vi "FTW-Container-Support-XML-LVSchemaToIR.vi"(0 "XML Node":refnum<k20>, 5 "Indent Characters":string, 7 "Indent Level":i32=1, 11 "error in":errorcluster) -> (4 "XML Node out":refnum<k20>, 6 "Serialized Node":string, 15 "error out":errorcluster)   [LabVIEW 2013, in "FTW-Container.lvclass"]
uses:
  FTW-Container.lvclass
  <resource>/objmgr/DOMUserDefRef.rc
panel:
  # "Inputs"
  # "Outputs"
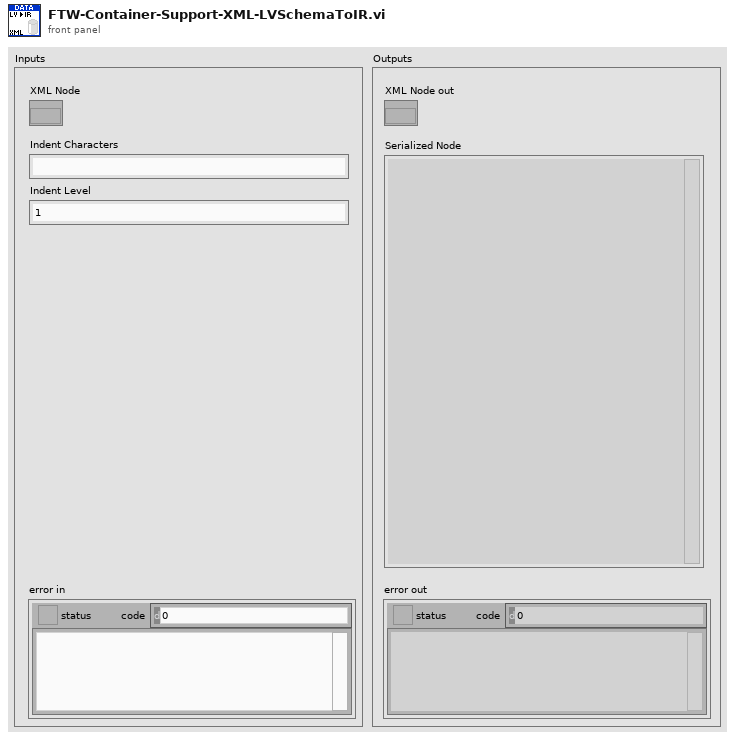
[diagram p1: front panel]
types:
  T1 = typedef "FTW-JSON-Datatype.ctl" = enum16{"Object", "Array", "String", "Number", "Boolean", "NULL", "<Refnum>", "<Enum>", "<Unknown>"}
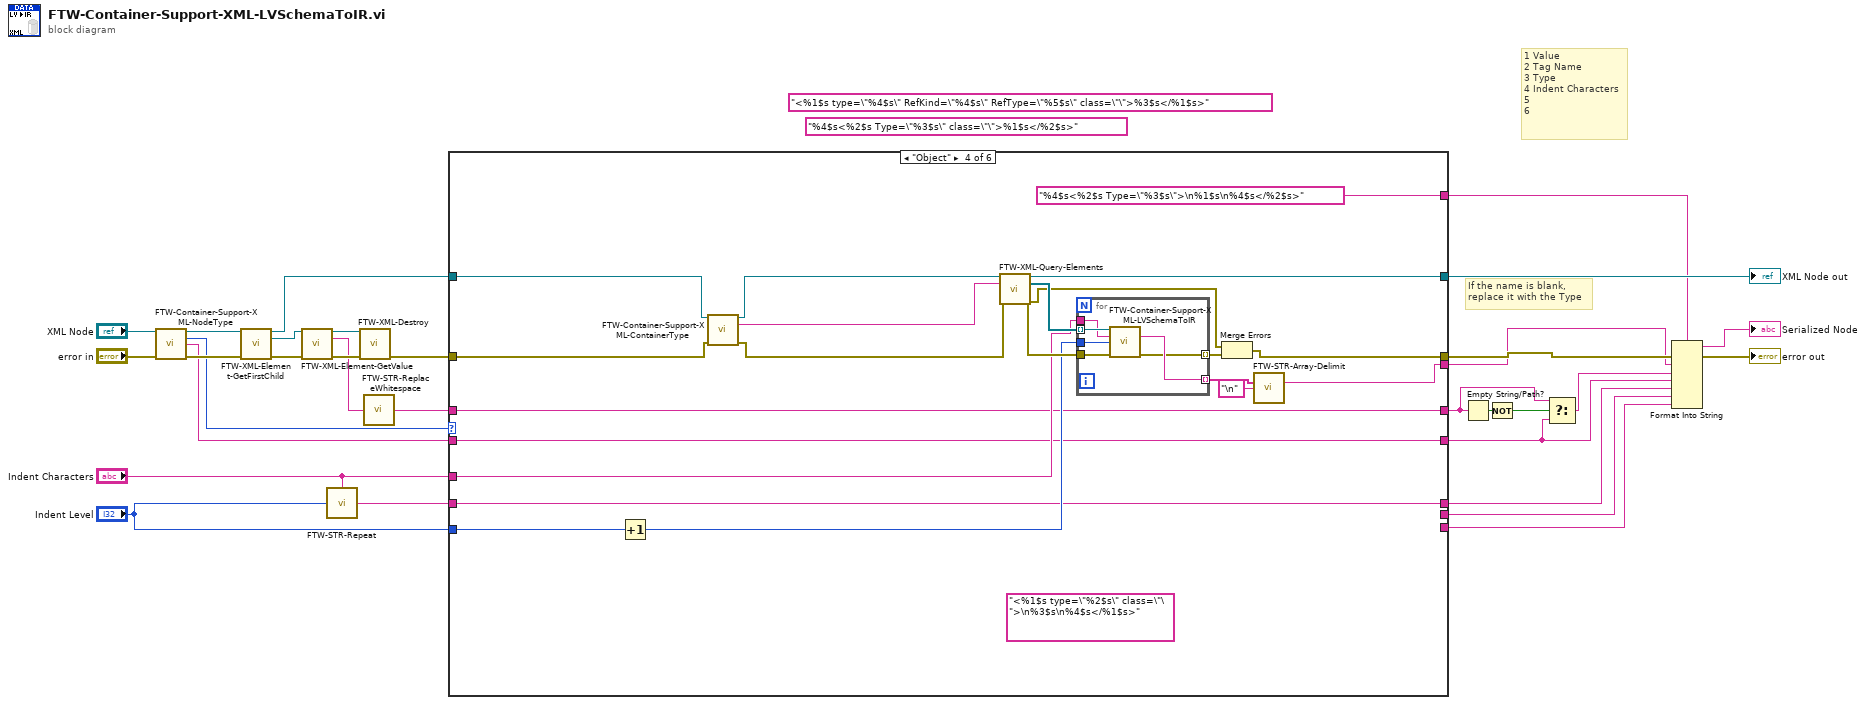
[diagram p0: block diagram]
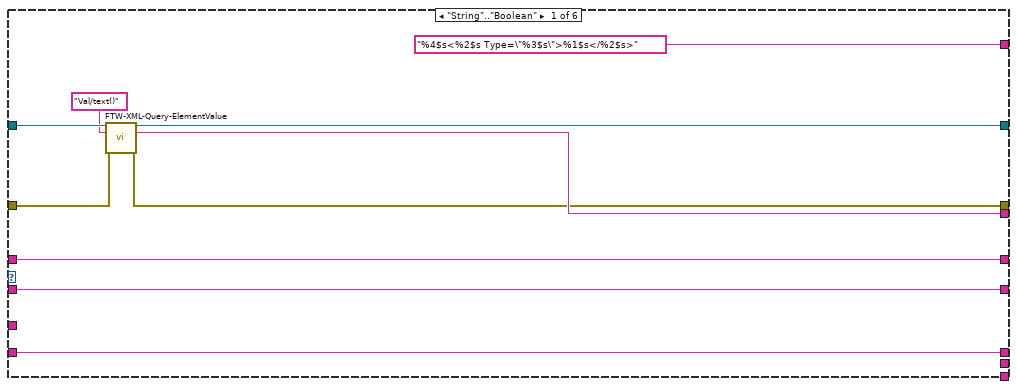
[diagram p2: hidden frame]
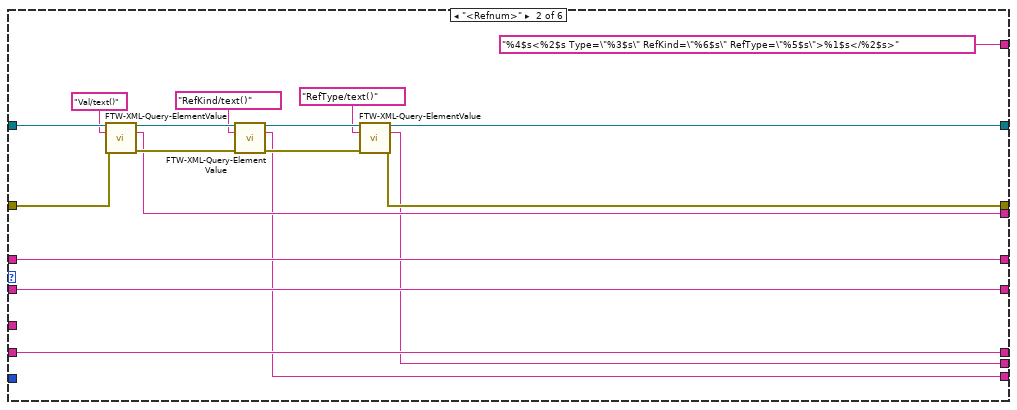
[diagram p3: hidden frame]
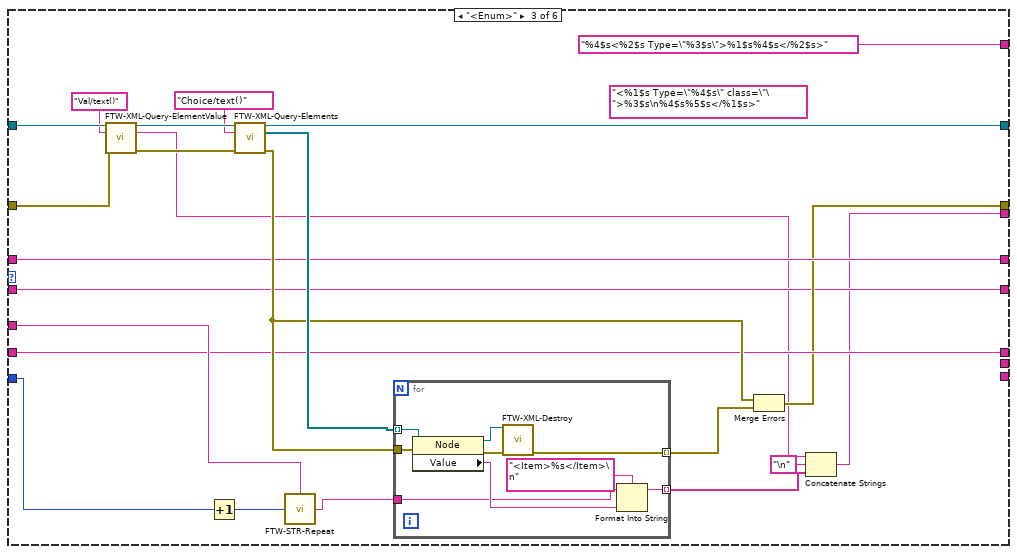
[diagram p4: hidden frame]
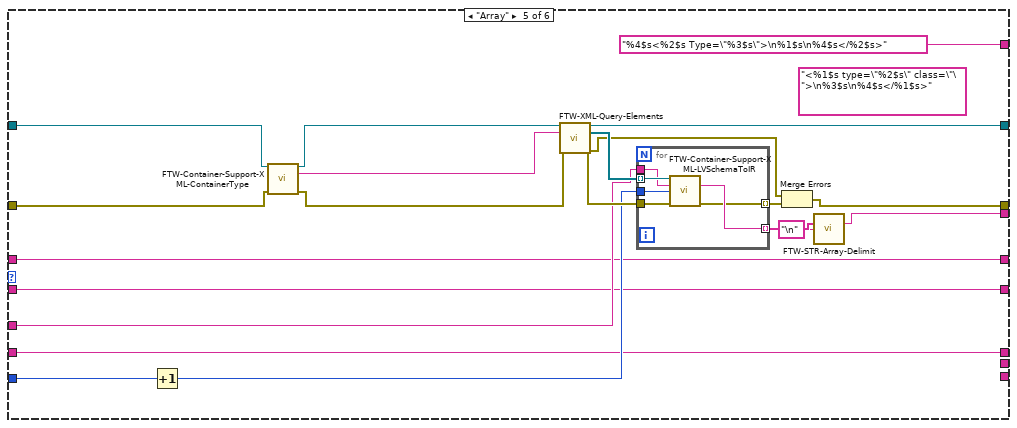
[diagram p5: hidden frame]
diagram:
  (unwired) "%4$s<%2$s Type=\"%3$s\" class=\"\">%1$s</%2$s>"
  (unwired) "<%1$s type=\"%4$s\" RefKind=\"%4$s\" RefType=\"%5$s\" class=\"\">%3$s</%1$s>" ("format string")
  # "If the name is blank,\nreplace it with the Type"
  # "1 Value\n2 Tag Name\n3 Type\n4 Indent Characters\n5\n6"
  n1 = call "FTW-Container-Support-XML-NodeType.vi"("Element Node"="XML Node", "error in"="error in") -> ("Element Node out"=w23:refnum<k20>, "JSON Type"=w20:T1, "Node XML Type"=w12:string, "error out"=w21:errorcluster)  [unwired: 10 in]
  n2 = call "FTW-XML-Element-GetFirstChild.vi"("Element Node"=w23, "error in"=w21) -> ("Element Node out"=w26:refnum<k20>, "First Child Element Node"=w27:refnum<k20>, "error out"=w28:errorcluster)  [unwired: 10 in, 1 out]
  n3 = call "FTW-XML-Element-GetValue.vi"("XML Node"=w27, "error in"=w28) -> ("XML Node out"=w30:refnum<k20>, "Node Text Value"=w17:string, "error out"=w31:errorcluster)  [unwired: 11 in]
  n4 = call "FTW-STR-Repeat.vi"("Times to Repeat"="Indent Level", "String to Repeat"="Indent Characters") -> ("Indented String"=w13:string)
  n5 = call "FTW-XML-Destroy.vi"("XML Node"=w30, "error in"=w31) -> ("error out"=w29:errorcluster)  [unwired: 13 in]
  n6 = call "FTW-STR-ReplaceWhitespace.vi"("Input"=w17) -> ("Output"=w14:string)  [unwired: 3 in]
  n7 = case shown="\"Object\"" w20 {
    tunnel: "Indent Characters" -> [_ _ w69 w105 w131 _]
    tunnel: w29 -> [w41 w59 w82 w99 w125 w145]
    tunnel: w14 -> [w36 w49 w66 w94 w121 _]
    tunnel: [w34 w48 w65 w97 w123 w145] -> w2
    tunnel: w26 -> [w40 w58 w81 w101 w127 w144]
    tunnel: [w39 w52 w76 w109 w135 w144] -> w25
    tunnel: w12 -> [w32 w46 w64 w93 w120 _]
    tunnel: w13 -> [w33 w47 w67 w92 w119 _]
    tunnel: "Indent Level" -> [_ _ w71 w104 w130 _]
    tunnel: ["%4$s<%2$s Type=\"%3$s\">%1$s</%2$s>" "%4$s<%2$s Type=\"%3$s\" RefKind=\"%6$s\" RefType=\"%5$s\">%1$s</%2$s>" "%4$s<%2$s Type=\"%3$s\">%1$s%4$s</%2$s>" "%4$s<%2$s Type=\"%3$s\">\n%1$s\n%4$s</%2$s>" "%4$s<%2$s Type=\"%3$s\">\n%1$s\n%4$s</%2$s>" _] -> w15
    tunnel: [w36 w49 w66 w94 w121 _] -> w9
    tunnel: [w35 w44 w62 w95 w122 _] -> w1
    tunnel: [w33 w47 w67 w92 w119 _] -> w6
    tunnel: [w32 w46 w64 w93 w120 _] -> w7
    tunnel: [_ w43 _ _ _ _] -> w5
    tunnel: [_ w42 _ _ _ _] -> w4
    frame "String".."Boolean" {
      n8 = call "FTW-XML-Query-ElementValue.vi"("XML Node"=w40, "XPath"="Val/text()", "error in"=w41) -> ("XML Node out"=w39:refnum<k20>, "Value"=w35:string, "error out"=w34:errorcluster)  [unwired: 9 in, 1 out]
    }
    frame "<Refnum>" {
      n9 = call "FTW-XML-Query-ElementValue.vi"("XML Node"=w58, "XPath"="Val/text()", "error in"=w59) -> ("XML Node out"=w56:refnum<k20>, "Value"=w44:string, "error out"=w54:errorcluster)  [unwired: 9 in, 1 out]
      n10 = call "FTW-XML-Query-ElementValue.vi"("XML Node"=w56, "XPath"="RefKind/text()", "error in"=w54) -> ("XML Node out"=w53:refnum<k20>, "Value"=w42:string, "error out"=w51:errorcluster)  [unwired: 9 in, 1 out]
      n11 = call "FTW-XML-Query-ElementValue.vi"("XML Node"=w53, "XPath"="RefType/text()", "error in"=w51) -> ("XML Node out"=w52:refnum<k20>, "Value"=w43:string, "error out"=w48:errorcluster)  [unwired: 9 in, 1 out]
    }
    frame "<Enum>" {
      (unwired) "<%1$s Type=\"%4$s\" class=\"\">%3$s\n%4$s%5$s</%1$s>" ("format string")
      n12 = call "FTW-XML-Query-ElementValue.vi"("XML Node"=w81, "XPath"="Val/text()", "error in"=w82) -> ("XML Node out"=w79:refnum<k20>, "Value"=w61:string, "error out"=w77:errorcluster)  [unwired: 9 in, 1 out]
      n13 = Increment(x=w71) -> (x+1=w70:i32)
      n14 = call "FTW-XML-Query-Elements.vi"("XML Node"=w79, "XPath Query"="Choice/text()", "error in"=w77) -> ("XML Node out"=w76:refnum<k20>, "Matching Nodes"=w75:refnum<k20>[], "error out"=w74:errorcluster)  [unwired: 9 in, 1 out]
      n15 = call "FTW-STR-Repeat.vi"("Times to Repeat"=w70, "String to Repeat"=w69) -> ("Indented String"=w68:string)
      n16 = for {
        tunnel: w75 -> [w91] mode=indexing
        tunnel: w74 -> [w90]
        tunnel: [w84] -> w72 mode=indexing
        tunnel: [w87] -> w73 mode=indexing
        tunnel: w68 -> [w83]
        n17 = property class="Node"(reference=w91, error in=w90) -> (reference out=w89:refnum<k20>, error out=w88:errorcluster, "Value"=w86:string)
        n18 = call "FTW-XML-Destroy.vi"("XML Node"=w89, "error in"=w88) -> ("error out"=w87:errorcluster)  [unwired: 13 in]
        n19 = Format Into String(format string="<Item>%s</Item>\n", initial string=w83, w86) -> (resulting string=w84:string)  [unwired: 1 in, 1 out]
      }
      n20 = Merge Errors(w74, w73) -> (w65:errorcluster)
      n21 = Concatenate Strings(w61, "\n" ("string"), w72) -> (w62:string)
    }
    frame "Object" {
      (unwired) "<%1$s type=\"%2$s\" class=\"\">\n%3$s\n%4$s</%1$s>" ("format string")
      n22 = Increment(x=w104) -> (x+1=w103:i32)
      n23 = call "FTW-Container-Support-XML-ContainerType.vi"("Element Node"=w101, "error in"=w99) -> ("Element Node out"=w100:refnum<k20>, "Parent XPath Query"=w102:string, "error out"=w98:errorcluster)  [unwired: 9 in, 2 out]
      n24 = call "FTW-XML-Query-Elements.vi"("XML Node"=w100, "XPath Query"=w102, "error in"=w98) -> ("XML Node out"=w109:refnum<k20>, "Matching Nodes"=w111:refnum<k20>[], "error out"=w108:errorcluster)  [unwired: 9 in, 1 out]
      n25 = for {
        tunnel: w108 -> [w117]
        tunnel: w111 -> [w116] mode=indexing
        tunnel: [w115] -> w107 mode=indexing
        tunnel: [w114] -> w110 mode=indexing
        tunnel: w103 -> [w113]
        tunnel: w105 -> [w112]
        n26 = call "FTW-Container-Support-XML-LVSchemaToIR.vi"("XML Node"=w116, "Indent Characters"=w112, "Indent Level"=w113, "error in"=w117) -> ("Serialized Node"=w115:string, "error out"=w114:errorcluster)  [unwired: 9 in, 1 out]
      }
      n27 = Merge Errors(w108, w110) -> (w97:errorcluster)
      n28 = call "FTW-STR-Array-Delimit.vi"("Array of Strings"=w107, "Delimiter"="\n") -> ("Delimited String"=w95:string)  [unwired: 13 in]
    }
    frame "Array" {
      (unwired) "<%1$s type=\"%2$s\" class=\"\">\n%3$s\n%4$s</%1$s>" ("format string")
      n29 = Increment(x=w130) -> (x+1=w129:i32)
      n30 = call "FTW-Container-Support-XML-ContainerType.vi"("Element Node"=w127, "error in"=w125) -> ("Element Node out"=w126:refnum<k20>, "Parent XPath Query"=w128:string, "error out"=w124:errorcluster)  [unwired: 9 in, 2 out]
      n31 = call "FTW-XML-Query-Elements.vi"("XML Node"=w126, "XPath Query"=w128, "error in"=w124) -> ("XML Node out"=w135:refnum<k20>, "Matching Nodes"=w137:refnum<k20>[], "error out"=w134:errorcluster)  [unwired: 9 in, 1 out]
      n32 = for {
        tunnel: w134 -> [w143]
        tunnel: w137 -> [w142] mode=indexing
        tunnel: [w141] -> w133 mode=indexing
        tunnel: [w140] -> w136 mode=indexing
        tunnel: w129 -> [w139]
        tunnel: w131 -> [w138]
        n33 = call "FTW-Container-Support-XML-LVSchemaToIR.vi"("XML Node"=w142, "Indent Characters"=w138, "Indent Level"=w139, "error in"=w143) -> ("Serialized Node"=w141:string, "error out"=w140:errorcluster)  [unwired: 9 in, 1 out]
      }
      n34 = Merge Errors(w134, w136) -> (w123:errorcluster)
      n35 = call "FTW-STR-Array-Delimit.vi"("Array of Strings"=w133, "Delimiter"="\n") -> ("Delimited String"=w122:string)  [unwired: 13 in]
    }
    frame "NULL", "<Unknown>" {
    }
  }
  "XML Node out" <- w25
  n36 = Empty String/Path?(string/path=w9) -> (empty?=w10:bool)
  n37 = Not(x=w10) -> (.not. x?=w3:bool)
  n38 = Select(t=w9, s=w3, f=w7) -> (s? t:f=w8:string)
  n39 = Format Into String(format string=w15, error in=w2, w1, w8, w7, w6, w5, w4) -> (resulting string=→"Serialized Node":string, error out=→"error out":errorcluster)  [unwired: 1 in]
